vi "TestConfig.vi"(8 "ErrorIn Array":errorcluster[](array[cluster])) -> (0 "ErrorOut Array":errorcluster[](array[cluster]), 3 "PSW Out":bool)   [LabVIEW 2018]
doc: "This VI allows the user decide wether to enable automatic error handling and leave the python script command window open to aid in debuging."
uses:
  <userlib>/NIST/NISTErrorLib/NISTErrorLib.lvlib
panel:
  in  "Stop Button":bool
  in  "PSW In":bool
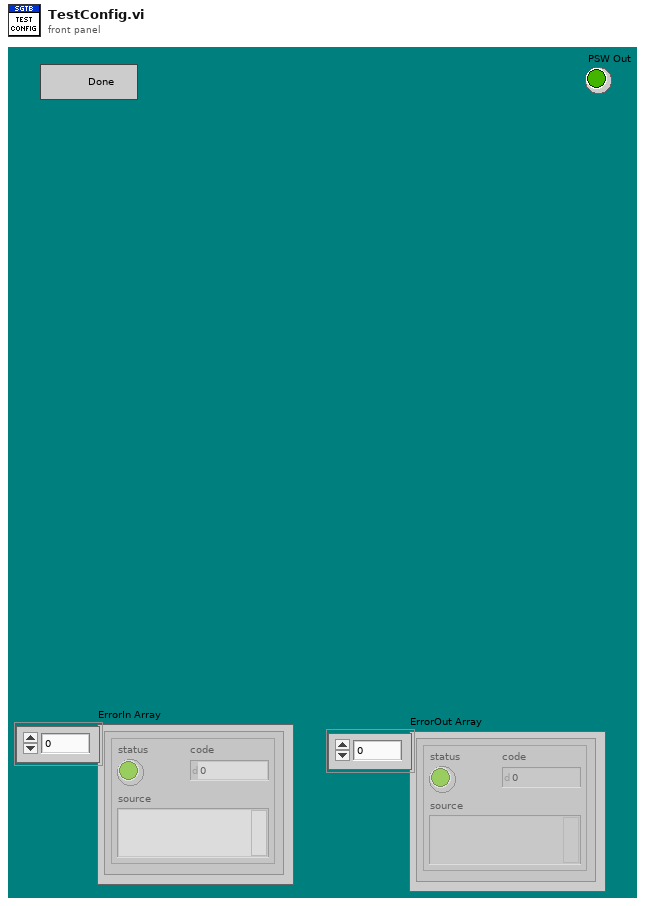
[diagram p1: front panel]
types:
  T1 = enum32{"Invalid", "Standard", "Closed", "Hidden", "Minimized", "Maximized"}
  T2 = enum32{"Invalid", "Default", "Floating", "Floating/Auto-Hide", "Modal"}
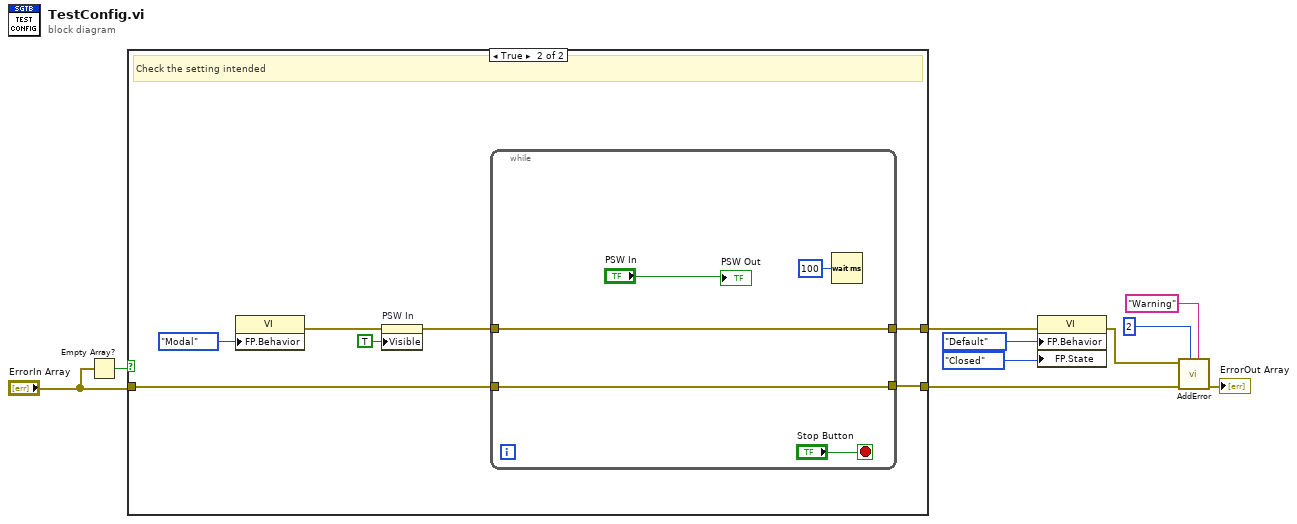
[diagram p0: block diagram]
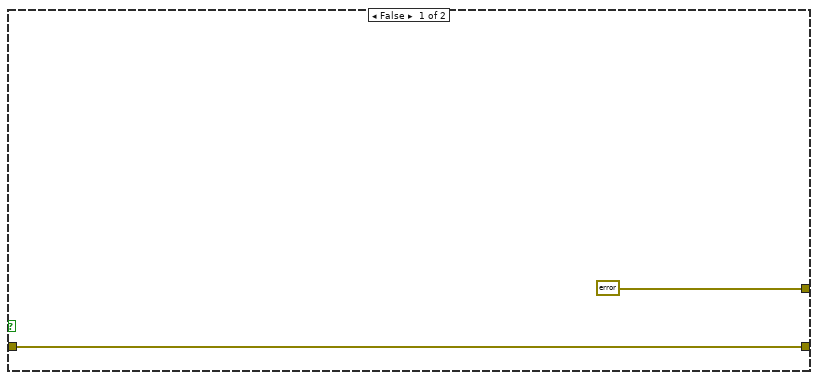
[diagram p2: hidden frame]
diagram:
  n1 = Empty Array?(array="ErrorIn Array") -> (empty?=w10:bool)
  n2 = case shown="True" w10 {
    tunnel: "ErrorIn Array" -> [w12 w18]
    tunnel: [w12 w16] -> w1
    tunnel: [errorcluster {"status"=FALSE, "code"=0, "source"=""} ("error out") w17] -> w3
    frame False {
    }
    frame True {
      # "Check the setting intended"
      n3 = property class="VI"("FP.Behavior"=T2."Modal" ("Front Panel Window:Behavior")) -> (error out=w15:errorcluster)  [unwired: 2 in, 1 out]
      n4 = property on="PSW In" class="Bool (strict)"(error in=w15, "Visible"=TRUE) -> (error out=w14:errorcluster)  [unwired: 1 in, 1 out]
      n5 = while {
        tunnel: w18 -> [w22]
        tunnel: w14 -> [w23]
        tunnel: [w23] -> w17
        tunnel: [w22] -> w16
        stop <- "Stop Button" stop-if-true
        n6 = Wait (ms)(milliseconds to wait=u32 100) -> ()  [unwired: 1 out]
        "PSW Out" <- "PSW In"
      }
    }
  }
  n7 = property class="VI"(error in=w3, "FP.Behavior"=T2."Default" ("Front Panel Window:Behavior"), "FP.State"=T1."Closed" ("Front Panel Window:State")) -> (error out=w8:errorcluster)  [unwired: 1 in, 1 out]
  n8 = call <userlib>:"AddError.vi"("Severity"="Warning", "Priority"=u8 2, "ErrorArray"=w1, "error in (no error)"=w8) -> ("ErrorArray"=→"ErrorOut Array":errorcluster[])  [unwired: 6 in, 1 out]
